vi "ErrorDrawerSettingsFGV.vi"(7 "Get or Set (Get)":T1, 8 "Error In":errorcluster, 11 "Error structure drawer settings":T2={"Error control config"={"Error control path"=path "", "Error indicator path"=path "", "Error control vertical spacing from existing FP items"=0, "Error-control to error-indicator horizontal spacing on FP"=0, "Error control vertical spacing from existing BD items"=0, "Error indicator vertical spacing from existing BD items"=0}, "BD alignment settings"={"Controls"=enum."Top Edges", "Indicators"=enum."Top Edges"}, "Case structure outer whitespace (px)"={"Control terminals right-side"=0, "Indicator terminals left-side"=0}, "Case structure inner whitespace (px)"={"Left"=0, "Right"=0, "Top"=0, "Bottom"=0}, "Case structure constants"={"Border thickness"=0, "Case-menu height"=0, "Half height/width of a tunnel"=4}, "CS size if BD is empty"={"Width (%)"=70.0, "Height (%)"=50.0}, "Control constants"={"Half-height of terminal"=8}}) -> (0 "Error Out":errorcluster, 3 "Error structure drawer settings":T2={"Error control config"={"Error control path"=path "", "Error indicator path"=path "", "Error control vertical spacing from existing FP items"=40, "Error-control to error-indicator horizontal spacing on FP"=40, "Error control vertical spacing from existing BD items"=10, "Error indicator vertical spacing from existing BD items"=10}, "BD alignment settings"={"Controls"=enum."Left Edges", "Indicators"=enum."Left Edges"}, "Case structure outer whitespace (px)"={"Control terminals right-side"=10, "Indicator terminals left-side"=10}, "Case structure inner whitespace (px)"={"Left"=20, "Right"=20, "Top"=20, "Bottom"=40}, "Case structure constants"={"Border thickness"=6, "Case-menu height"=16, "Half height/width of a tunnel"=4}, "CS size if BD is empty"={"Width (%)"=70.0, "Height (%)"=50.0}, "Control constants"={"Half-height of terminal"=8}})   [LabVIEW 2017, in "ErrorStructureDrawer.lvlib"]
doc: "FGV that can store or retrieve the configuration settings for the error structure drawer."
uses:
  ErrorStructureDrawer.lvlib
  Controls/ErrorStructureDrawerSettings.ctl
  Controls/ErrorControlConfig.ctl
  Controls/BD_AlignmentSettings.ctl
  Controls/CaseStructureOuterWhitespace.ctl
  Controls/CaseStructureInnerWhitespace.ctl
  Controls/CaseStructureConstants.ctl
  Controls/CaseStructureSizeIfBD_Empty.ctl
  Controls/ControlConstants.ctl
  Controls/GetSetCommand.ctl
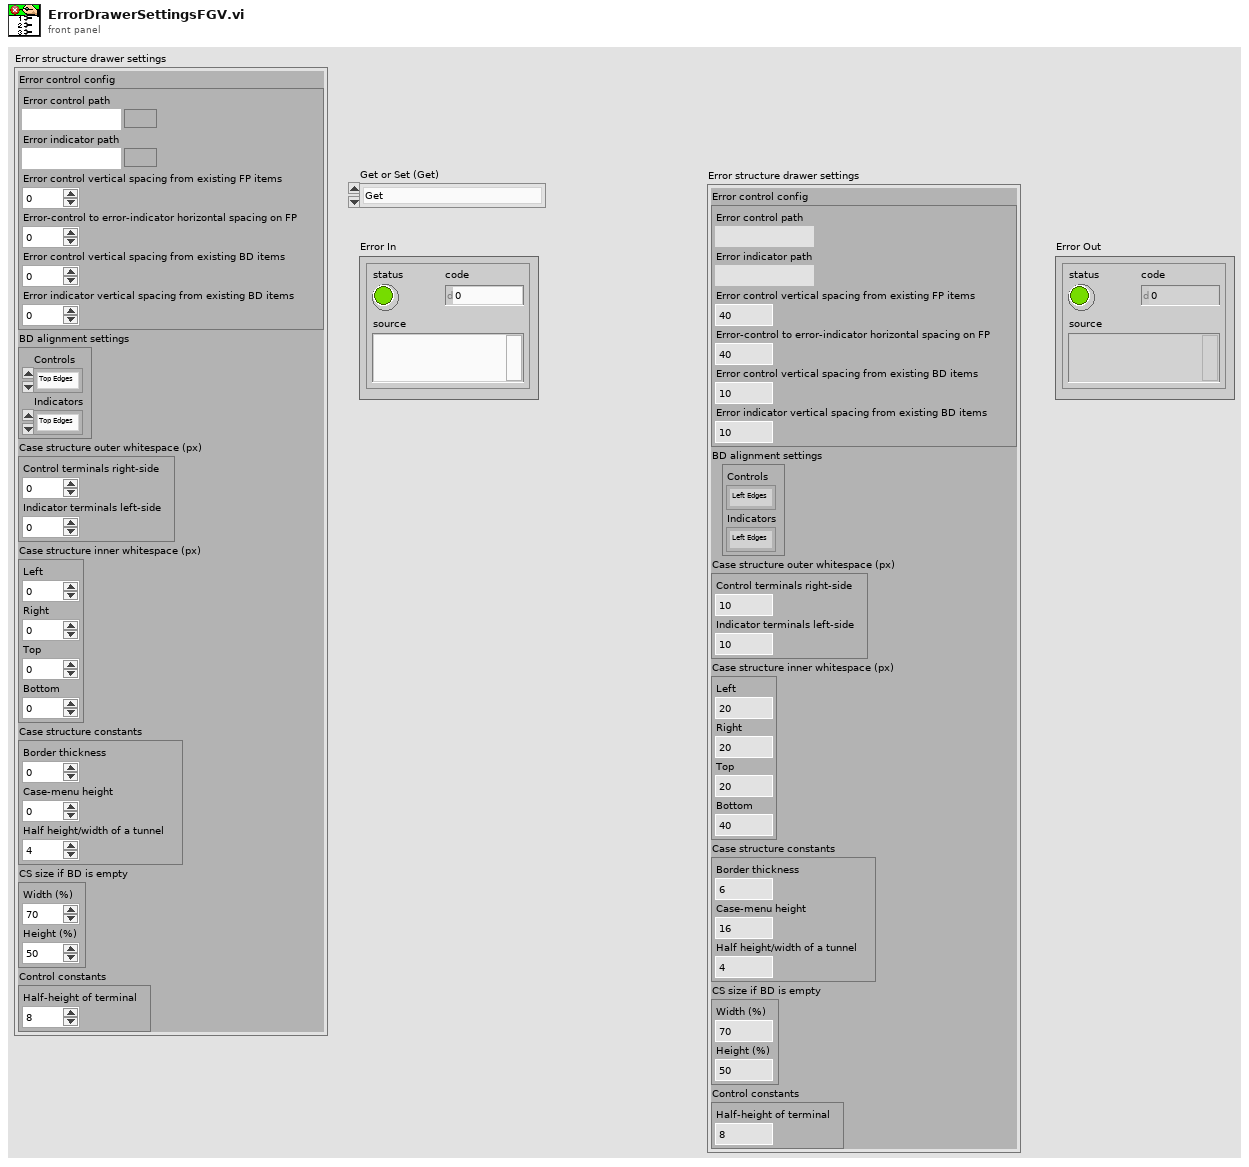
[diagram p1: front panel]
types:
  T1 = typedef "ErrorStructureDrawer.lvlib/GetSetCommand.ctl" = enum16{"Get", "Set"}
  T2 = typedef "ErrorStructureDrawer.lvlib/ErrorStructureDrawerSettings.ctl" = cluster{"Error control config":T3, "BD alignment settings":T4, "Case structure outer whitespace (px)":T5, "Case structure inner whitespace (px)":T6, "Case structure constants":T7, "CS size if BD is empty":T8, "Control constants":T9}
  T3 = typedef "ErrorStructureDrawer.lvlib/ErrorControlConfig.ctl" = cluster{"Error control path":path, "Error indicator path":path, "Error control vertical spacing from existing FP items":i16, "Error-control to error-indicator horizontal spacing on FP":i16, "Error control vertical spacing from existing BD items":i32, "Error indicator vertical spacing from existing BD items":i32}
  T4 = typedef "ErrorStructureDrawer.lvlib/BD_AlignmentSettings.ctl" = cluster{"Controls":enum32{"Top Edges", "Vertical Centers", "Bottom Edges", "Left Edges", "Horizontal Centers", "Right Edges"}, "Indicators":enum32{"Top Edges", "Vertical Centers", "Bottom Edges", "Left Edges", "Horizontal Centers", "Right Edges"}}
  T5 = typedef "ErrorStructureDrawer.lvlib/CaseStructureOuterWhitespace.ctl" = cluster{"Control terminals right-side":i32, "Indicator terminals left-side":i32}
  T6 = typedef "ErrorStructureDrawer.lvlib/CaseStructureInnerWhitespace.ctl" = cluster{"Left":u32, "Right":u32, "Top":u32, "Bottom":u32}
  T7 = typedef "ErrorStructureDrawer.lvlib/CaseStructureConstants.ctl" = cluster{"Border thickness":u32, "Case-menu height":u32, "Half height/width of a tunnel":i32}
  T8 = typedef "ErrorStructureDrawer.lvlib/CaseStructureSizeIfBD_Empty.ctl" = cluster{"Width (%)":dbl, "Height (%)":dbl}
  T9 = typedef "ErrorStructureDrawer.lvlib/ControlConstants.ctl" = cluster{"Half-height of terminal":i32}
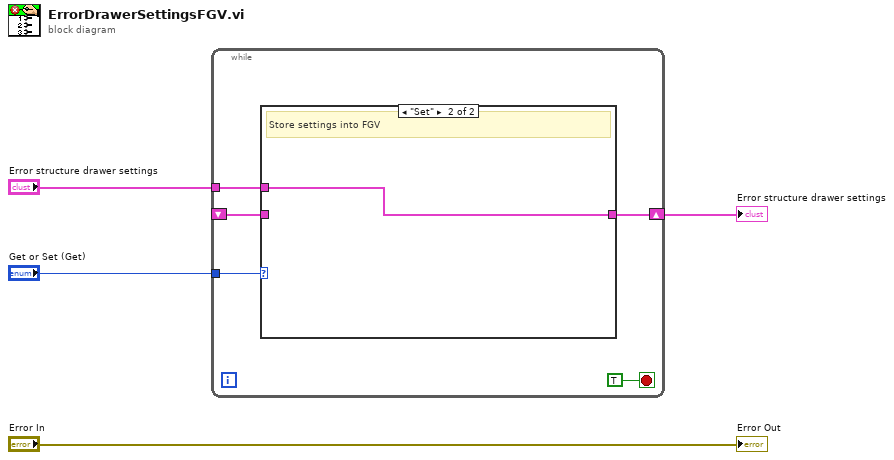
[diagram p0: block diagram]
diagram:
  n1 = while {
    shift-right: [w9] -> w3
    shift-left: _ -> [w7]
    tunnel: "Error structure drawer settings" -> [w8]
    tunnel: "Get or Set (Get)" -> [w5]
    stop <- TRUE stop-if-true
    n2 = case shown="\"Set\"" w5 {
      tunnel: [w10 w11] -> w9
      tunnel: w8 -> [_ w11]
      tunnel: w7 -> [w10 _]
      frame "Get" {
        # "Retrieve settings from FGV"
      }
      frame "Set" {
        # "Store settings into FGV"
      }
    }
  }
  "Error structure drawer settings" <- w3
  "Error Out" <- "Error In"
